vi "RSZVB Trace Export Data With Options.vi"(6 "Export Format (0: Unformatted)":i32(ring) items=["Unformatted", "Formatted"], 7 "Export Data (0: Complex Values)":i32(ring) items=["Complex Values", "Linear magnitude and phase", "dB-magnitude and phase"], 8 "error in (no error)":errorcluster {"code" format="%.0x"}, 9 "File Name (Trc1.s1p)":string="Trc1.s1p", 10 "Trace Name (Trc1)":string="Trc1", 11 "VISA session":refnum<visa-resource-name>) -> (0 "error out":errorcluster {"code" format="%.0x"}, 3 "dup VISA session":refnum<visa-resource-name>)   [LabVIEW 2011]
doc: "This VI stores the trace data of a specified trace to a trace file.\n\nNote(s):\n\nTraces are created using the CALCulte<Ch>:PARameter:SDEFine... command.\n\n*.s<n>p touchstone files (<n> = 2, 3, 4) are intended for a complete set of <n>-port S-parameters. Data export fails if the active channel does not contain the full set of <n>^2 traces. If the necessary trace are available, '<trc_name>' can be the name of any of the traces.\n\nRemote-control command(s):\nMMEMory:STORe:TRACe '<trc_name>','<file_name>'[,UNFormatted | FORMatted, COMPlex | LINPhase | LOGPhase]"
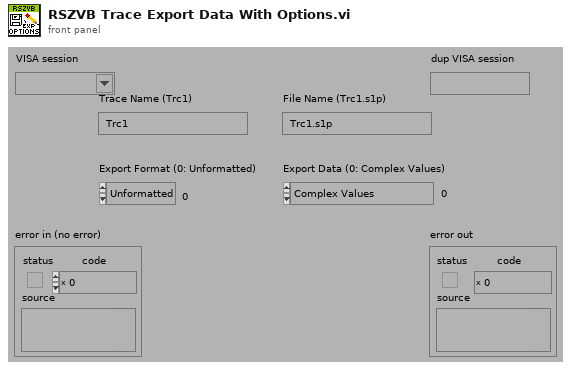
[diagram p1: front panel]
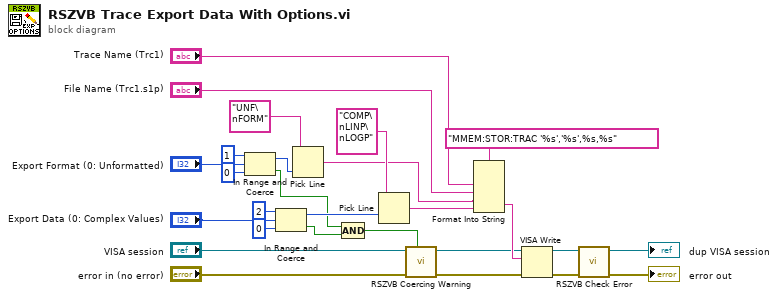
[diagram p0: block diagram]
diagram:
  n1 = In Range and Coerce(upper limit=1, x="Export Format (0: Unformatted)", lower limit=0) -> (coerced(x)=w9:i32, In Range?=w5:bool)
  n2 = In Range and Coerce(upper limit=2, x="Export Data (0: Complex Values)", lower limit=0) -> (coerced(x)=w8:i32, In Range?=w6:bool)
  n3 = Pick Line(multi-line string="UNF\nFORM", line index=w9) -> (output string=w16:string)  [unwired: 1 in]
  n4 = Compound Arithmetic op=AND(w5, w6) -> (w7:bool)
  n5 = Pick Line(multi-line string="COMP\nLINP\nLOGP", line index=w8) -> (output string=w17:string)  [unwired: 1 in]
  n6 = call "RSZVB Coercing Warning.vi"("In Range?"=w7, "error in (no error)"="error in (no error)", "VISA session"="VISA session") -> ("error out"=w3:errorcluster, "dup VISA session"=w4:refnum<visa-resource-name>)  [unwired: 7 in]
  n7 = Format Into String(format string="MMEM:STOR:TRAC '%s','%s',%s,%s", "Trace Name (Trc1)", "File Name (Trc1.s1p)", w16, w17) -> (resulting string=w24:string)  [unwired: 2 in, 1 out]
  n8 = VISA Write(VISA resource name=w4, write buffer=w24, error in (no error)=w3) -> (VISA resource name out=w25:refnum<visa-resource-name>, error out=w26:errorcluster)  [unwired: 1 out]
  n9 = call "RSZVB Check Error.vi"("error in (no error)"=w26, "VISA session"=w25) -> ("error out"=→"error out":errorcluster, "dup VISA session"=→"dup VISA session":refnum<visa-resource-name>)  [unwired: 8 in]
